vi "Test Program single core.vi"(0 "DataMemory/Fxp":dbl[](array[numeric])=[0.0, 3.0, 2.0, 3.0, 4.0, 5.0, 9.0, 7.0, 42.0, 9.0, -1.0, 11.0, 15.0, 16.0, 17.0, 18.0, 19.0, 20.0, 0.0, 0.0, 0.0, 0.0, 0.0, 0.0, 0.0, 0.0, 0.0, 0.0, 0.0, 0.0, 0.0, 0.0, 0.0, 0.0, 0.0, 0.0, 0.0, 0.0, 0.0, 0.0, 0.0, 0.0, 0.0, 0.0, 0.0, 0.0, 0.0, 0.0, 0.0, 0.0, 0.0, 0.0, 0.0, 0.0, 0.0, 0.0, 0.0, 0.0, 0.0, 0.0, 0.0, 0.0, 0.0, 0.0, 0.0, 0.0, 0.0, 0.0, 0.0, 0.0, 0.0, 0.0, 0.0, 0.0, 0.0, 0.0, 0.0, 0.0, 0.0, 0.0, 0.0, 0.0, 0.0, 0.0, 0.0, 0.0, 0.0, 0.0, 0.0, 0.0, 0.0, 0.0, 0.0, 0.0, 0.0, 0.0, 0.0, 0.0, 0.0, 0.0, 0.0, 0.0, 0.0, 0.0, 0.0, 0.0, 0.0, 0.0, 0.0, 0.0, 0.0, 0.0, 0.0, 0.0, 0.0, 0.0, 0.0, 0.0, 0.0, 0.0, 0.0, 0.0, 0.0, 0.0, 0.0, 0.0, 0.0, 0.0, 0.0, 0.0, 0.0, 0.0, 0.0, 0.0, 0.0, 0.0, 0.0, 0.0, 0.0, 0.0, 0.0, 0.0, 0.0, 0.0, 0.0, 0.0, 0.0, 0.0, 0.0, 0.0, 0.0, 0.0, 0.0, 0.0, 0.0, 0.0, 0.0, 0.0, 0.0, 0.0, 0.0, 0.0, 0.0, 0.0, 0.0, 0.0, 0.0, 0.0, 0.0, 0.0, 0.0, 0.0, 0.0, 0.0, 0.0, 0.0, 0.0, 0.0, 0.0, 0.0, 0.0, 0.0, 0.0, 0.0, 0.0, 0.0, 0.0, 0.0, 0.0, 0.0, 0.0, 0.0, 0.0, 0.0, 0.0, 0.0, 0.0, 0.0, 0.0, 0.0, 0.0, 0.0, 0.0, 0.0, 0.0, 0.0, 0.0, 0.0, 0.0, 0.0, 0.0, 0.0, 0.0, 0.0, 0.0, 0.0, 0.0, 0.0, 0.0, 0.0, 0.0, 0.0, 0.0, 0.0, 0.0, 0.0, 0.0, 0.0, 0.0, 0.0, 0.0, 0.0, 0.0, 0.0, 0.0, 0.0, 0.0, 0.0, 0.0, 0.0, 0.0, 0.0, 0.0, 0.0, 0.0, 0.0, 0.0, 0.0, 0.0, 0.0, 0.0, 0.0, 0.0, 0.0, 0.0], 1 "CodeLine":T1={"Ex.Command"=enum."None", "Ex.AddressIn1"=0.0, "Ex.AddressIn2"=0.0, "WB.Command"=enum."In", "WB.AddressOut"=0.0, "Bypass1"=0.0, "Bypass 2"=0.0}) -> (8 "Data":dbl=5.0, 9 "Address":dbl=4.0)   [LabVIEW 2016]
uses:
  Z:/LiSARD_Reference_Project/Multicore_1.6beta/CodeConverter/Controls/CommandLine.ctl
  Z:/LiSARD_Reference_Project/Multicore_1.6beta/CodeConverter/Controls/EX.Command.ctl
  Z:/LiSARD_Reference_Project/Multicore_1.6beta/CodeConverter/Controls/WB.Operation.ctl
  Z:/LiSARD_Reference_Project/Multicore_1.6beta/CodeConverter/SoftCoreCodeConverter.lvlib
panel:
  out "element 2":dbl=3.0
  out "element":dbl=2.0
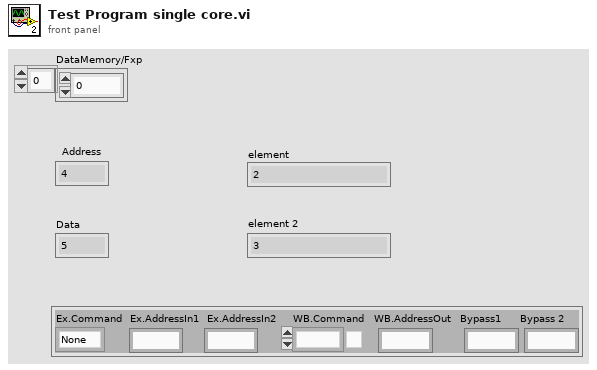
[diagram p1: front panel]
types:
  T1 = typedef "SoftCoreCodeConverter.lvlib/CommandLine.ctl" = cluster{"Ex.Command":T2, "Ex.AddressIn1":fxp<+,16,16>, "Ex.AddressIn2":fxp<+,16,16>, "WB.Command":T3, "WB.AddressOut":fxp<+,16,16>, "Bypass1":fxp<+,2,2>, "Bypass 2":fxp<+,2,2>}
  T2 = typedef "SoftCoreCodeConverter.lvlib/EX.Command.ctl" = enum8{"Default", "Sub", "None", "Fuse", "Abs", "AbsSub", "Const"}
  T3 = typedef "SoftCoreCodeConverter.lvlib/WB.Operation.ctl" = enum8{"In", "Out", "Mov", "Add", "Sub", "Mul", "Div", "None", "Sqr", "Sin", "Cos", "Sgl2Dbl", "Dbl2Int", "Int2Dbl", "Mlookup", "Dbl2Sgl", "G_IsPOS", "G_IsNEG", "G_IsNULL", "G_IsNNULL", "G_IsNAN", "G_IsNNAN", "G_IsIFTY", "G_IsNIFTY", "reserved_0", "reserved_1", "reserved_2", "reserved_3", "reserved_4", "reserved_5", "reserved_6", "reserved_7"}
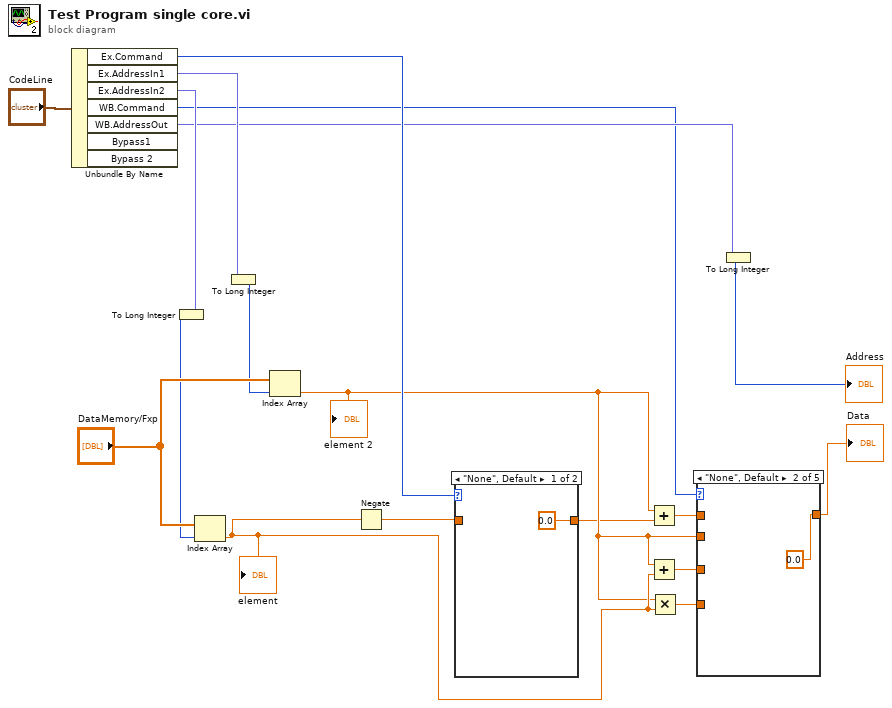
[diagram p0: block diagram]
diagram:
  n1 = Unbundle By Name("CodeLine") -> ("Ex.Command"=w16:T2, "Ex.AddressIn1"=w14:fxp<+,16,16>, "Ex.AddressIn2"=w12:fxp<+,16,16>, "WB.Command"=w9:T3, "WB.AddressOut"=w10:fxp<+,16,16>)  [unwired: 2 out]
  n2 = To Long Integer(number=w12) -> (32bit integer=w11:i32)
  n3 = Index Array "Index Array"(array="DataMemory/Fxp", index=w11) -> (element=w17:dbl)
  "element" <- w17
  n4 = To Long Integer(number=w14) -> (32bit integer=w13:i32)
  n5 = Index Array "Index Array"(array="DataMemory/Fxp", index=w13) -> (element=w15:dbl)
  "element 2" <- w15
  n6 = Negate(x=w17) -> (-x=w6:dbl)
  n7 = case shown="\"None\", Default" w16 {
    tunnel: w6 -> [_ w20]
    tunnel: [0.0 w20] -> w5
    frame "None", Default {
    }
    frame "Sub" {
    }
  }
  n8 = Add(x=w15, y=w5) -> (x+y=w4:dbl)
  n9 = Add(x=w15, y=w17) -> (x+y=w8:dbl)
  n10 = Multiply(x=w15, y=w17) -> (x*y=w7:dbl)
  n11 = case shown="\"None\", Default" w9 {
    tunnel: w8 -> [_ _ _ w24 _]
    tunnel: w7 -> [w21 _ _ _ _]
    tunnel: w15 -> [_ _ w23 _ _]
    tunnel: [w21 0.0 w23 w24 w25] -> w2
    tunnel: w4 -> [_ _ _ _ w25]
    frame "Mul" {
    }
    frame "None", Default {
    }
    frame "Mov" {
    }
    frame "Add" {
    }
    frame "Sub" {
    }
  }
  "Data" <- w2
  n12 = To Long Integer(number=w10) -> (32bit integer=→"Address":i32)
